vi "ROS_Topic_Write.vi"(2 "Msg in":string, 3 "ROS in":T1) -> (1 "ROS out":T1)   [LabVIEW 2010]
doc: "Prepends the length to Msg in before sending out the data on the specified topic. Use only for publishers and service clients. Messages need to be formatted using Message Building functionality. \n\nSetting Continuous to True will instruct the server to publish the message it received as quickly as possible, updating the message when a new ROS_Topic_Write is called."
uses:
  <userlib>/ROSforLV_0.1/ROS/Code/SubVIs/_ROSControl.ctl
  <userlib>/ROSforLV_0.1/ROS/Code/SubVIs/_ROSDirection.ctl
panel:
  in  "Continuous?":bool
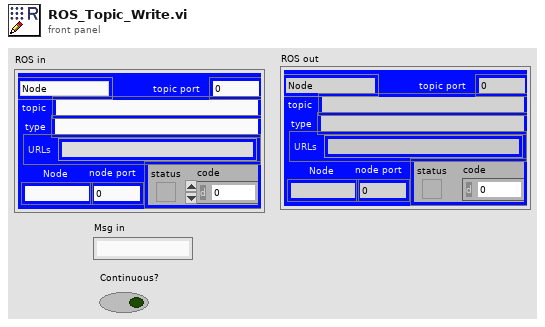
[diagram p1: front panel]
types:
  T1 = typedef "_ROSControl.ctl" = cluster{"topic port":u16, "Node":string, "topic":string, "type":string, "node port":u32, "error ":errorcluster, "Direction":T2, "APIs":string[]}
  T2 = typedef "_ROSDirection.ctl" = enum16{"Node", "Publisher", "Subscriber", "Service Client"}
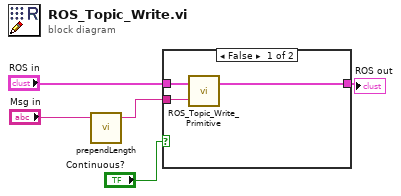
[diagram p0: block diagram]
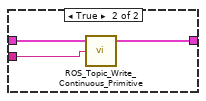
[diagram p2: hidden frame]
diagram:
  n1 = call <userlib>:"prependLength.vi"("msg in"="Msg in") -> ("msg out"=w2:string)  [unwired: 4 in]
  n2 = case shown="False" "Continuous?" {
    tunnel: "ROS in" -> [w8 w11]
    tunnel: [w7 w10] -> w4
    tunnel: w2 -> [w6 w9]
    frame False {
      n3 = call <userlib>:"ROS_Topic_Write_Primitive.vi"("Msg in"=w6, "ROS in"=w8) -> ("ROS out"=w7:T1)  [unwired: 1 in]
    }
    frame True {
      n4 = call <userlib>:"ROS_Topic_Write_Continuous_Primitive.vi"("Msg in"=w9, "ROS in"=w11) -> ("ROS out"=w10:T1)  [unwired: 3 in]
    }
  }
  "ROS out" <- w4
